vi "Config Process.vi"(8 "error in (no error)":errorcluster, 11 "View Model":T1) -> (0 "error out":errorcluster, 3 "View Model":T1)   [LabVIEW 2017]
doc: "Provides all functions for operates with data records (read/search/update)."
uses:
  View Model/Controls/View Model.ctl
  Error Handler/Controls/Error Model.ctl
  Error Handler/Controls/Error Data.ctl
  Error Handler/Controls/Error Type.ctl
  View Model/Controls/Shared Model.ctl
  Controls/Config Model.ctl
  Controls/Config CMD.ctl
  Controls/Config Data.ctl
  ATM Controller/Controls/Controller Model.ctl
  ATM Controller/Controls/Controller Overhead.ctl
  ATM Controller/Controls/Controller States.ctl
  ATM Controller/Controls/Controller Message Data.ctl
  ATM Controller/Controls/Controller Message Name.ctl
  ATM Controller/Controls/Controller CMD.ctl
  Views/User Console View/Controls/User Console - Transaction Enum.ctl
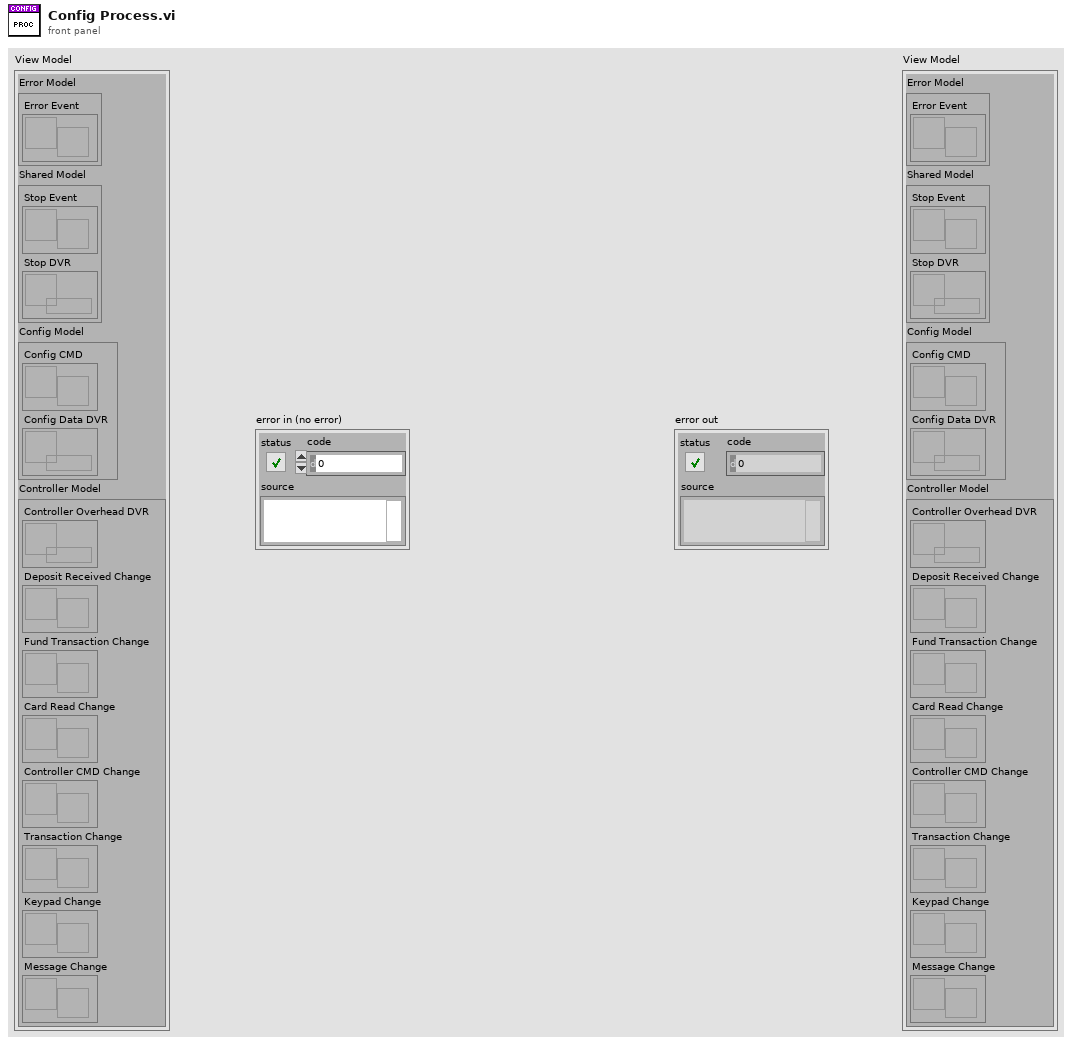
[diagram p1: front panel]
types:
  T1 = typedef "View Model.ctl" = cluster{"Error Model":T2, "Shared Model":T3, "Config Model":T4, "Controller Model":T5}
  T2 = typedef "Error Model.ctl" = cluster{"Error Event":refnum<user-event>}
  T3 = typedef "Shared Model.ctl" = cluster{"Stop Event":refnum<user-event>, "Stop DVR":refnum<data-value>}
  T4 = typedef "Config Model.ctl" = cluster{"Config CMD":refnum<user-event>, "Config Data DVR":refnum<data-value>}
  T5 = typedef "Controller Model.ctl" = cluster{"Controller Overhead DVR":refnum<data-value>, "Deposit Received Change":refnum<user-event>, "Fund Transaction Change":refnum<user-event>, "Card Read Change":refnum<user-event>, "Controller CMD Change":refnum<user-event>, "Transaction Change":refnum<user-event>, "Keypad Change":refnum<user-event>, "Message Change":refnum<user-event>}
  T6 = typedef "Config Data.ctl" = cluster{"Account Number":i32, "Balance":dbl, "First Name":string, "Last Name":string}
  T7 = typedef "Config CMD.ctl" = enum16{"Read", "Update", "Search"}
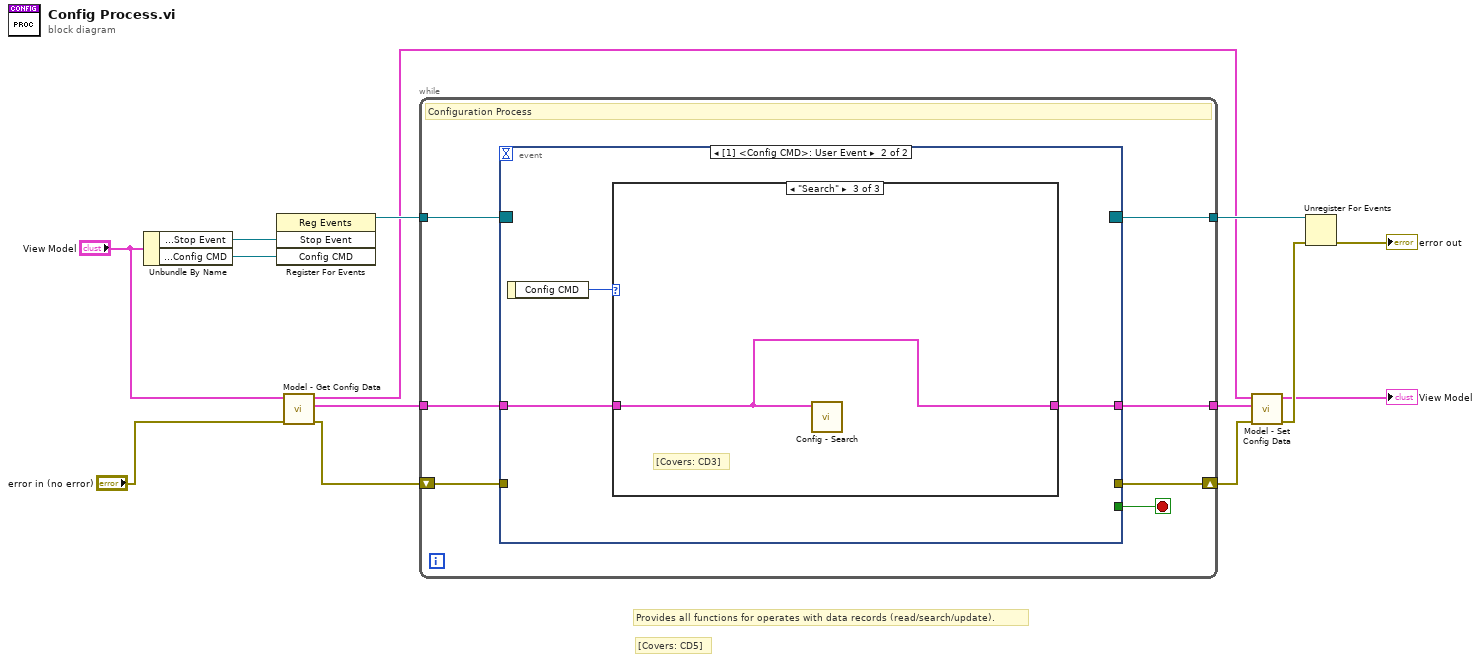
[diagram p0: block diagram]
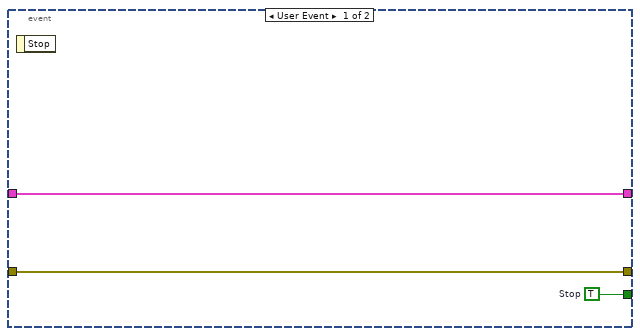
[diagram p2: hidden frame]
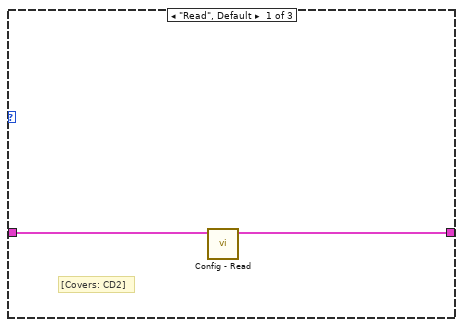
[diagram p3: hidden frame]
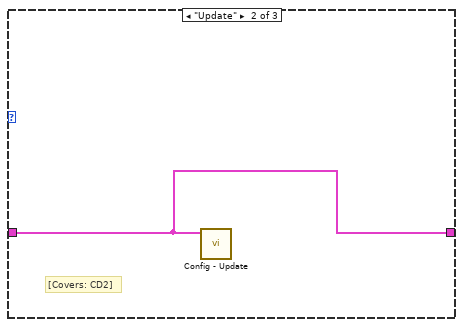
[diagram p4: hidden frame]
diagram:
  # "[Covers: CD5]"
  # "Provides all functions for operates with data records (read/search/update)."
  n1 = Unbundle By Name("View Model") -> ("Shared Model.Stop Event"=w14:refnum<user-event>, "Config Model.Config CMD"=w10:refnum<user-event>)
  n2 = register-events(w14, w10) -> (reference out=w13:refnum<event-registration>)  [unwired: 2 in, 1 out]
  n3 = call "Model - Get Config Data.vi"("error in (no error)"="error in (no error)", "View Model"="View Model") -> ("error out"=w7:errorcluster, "Config Data"=w6:T6, "View Model"=w3:T1)  [unwired: 7 in]
  n4 = while {
    tunnel: w13 -> [w21]
    shift-right: [w18] -> w4
    shift-left: w7 -> [w19]
    tunnel: [w17] -> w12
    tunnel: w6 -> [w16]
    tunnel: [w15] -> w5
    stop <- w20 stop-if-true
    # "Configuration Process"
    n5 = event shown="[1] <Config CMD>: User Event" {
      selector: w21 -> [_ _]
      dyn-events: [_ _] -> w17
      timeout: _ -> [_ _]
      tunnel: [w24 _] -> w20
      tunnel: w19 -> [w23 _]
      tunnel: [w23 _] -> w18
      tunnel: w16 -> [w22 w26]
      tunnel: [w22 w25] -> w15
      event User Event {
        w24 = TRUE  # Stop
        n6 = event-data() -> ()  [unwired: 1 in, 1 out]
      }
      event User Event {
        n7 = event-data() -> ("Config CMD"=w27:T7)  [unwired: 1 in]
        n8 = case shown="\"Search\"" w27 {
          tunnel: w26 -> [w29 w30 w31]
          tunnel: [w28 w30 w31] -> w25
          frame "Read", Default {
            # "[Covers: CD2]"
            n9 = call "Config - Read.vi"("Config Data"=w29) -> ("Config Data"=w28:T6)  [unwired: 9 in, 1 out]
          }
          frame "Update" {
            # "[Covers: CD2]"
            n10 = call "Config - Update.vi"("Config Data"=w30) -> ()  [unwired: 10 in, 1 out]
          }
          frame "Search" {
            # "[Covers: CD3]"
            n11 = call "Config - Search.vi"("Config Data"=w31) -> ()  [unwired: 8 in, 3 out]
          }
        }
      }
    }
  }
  n12 = call "Model - Set Config Data.vi"("error in (no error)"=w4, "Config Data"=w5, "View Model"=w3) -> ("error out"=w2:errorcluster, "View Model"=→"View Model":T1)  [unwired: 7 in]
  n13 = Unregister For Events(event registration refnum=w12, error in=w2) -> (error out=→"error out":errorcluster)
